vi "Insert Ramp Time Step Event.vi"(0 "VISA resource name":refnum<visa-resource-name>, 1 "Unit Address (1)":i16=1, 2 "Wait For Event (0: No)":u16(ring) items=["No", "Yes"], 5 "Current Step Number (1)":i16=1, 7 "Wait For Analog Inputs (0; 0; 0)":u16[](array[ring])=[0, 0, 0] items=["Don't Wait", "Wait For Analog Input"], 9 "Analog Input Values (32.0; 32.0; 32.0)":dbl[](array[numeric])=[32.0, 32.0, 32.0] format="%.2f", 11 "error in (no error)":errorcluster {"code" format="%.0x"}, 12 "Event Outputs (0; 0; 0; 0; 0; 0; 0; 0)":u16[](array[ring])=[0, 0, 0, 0, 0, 0, 0, 0] items=["Off", "On"], 13 "Wait For Event Inputs (0; 0; 0; 0)":u16[](array[ring])=[0, 0, 0, 0] items=["Don't Wait", "Wait For Off", "Wait For On"]) -> (4 "VISA resource name out":refnum<visa-resource-name>, 15 "error out":errorcluster {"code" format="%.0x"})   [LabVIEW 2010]
doc: "This is first part of two VIs, that inserts Ramp Time Step. This VI sets event inputs and outputs.\n\nNote: For correct function VIs MUST be activated in this sequence:\n1. WLF4 Insert Ramp Time Step Event.vi\n2. WLF4 Insert Ramp Time Step.vi"
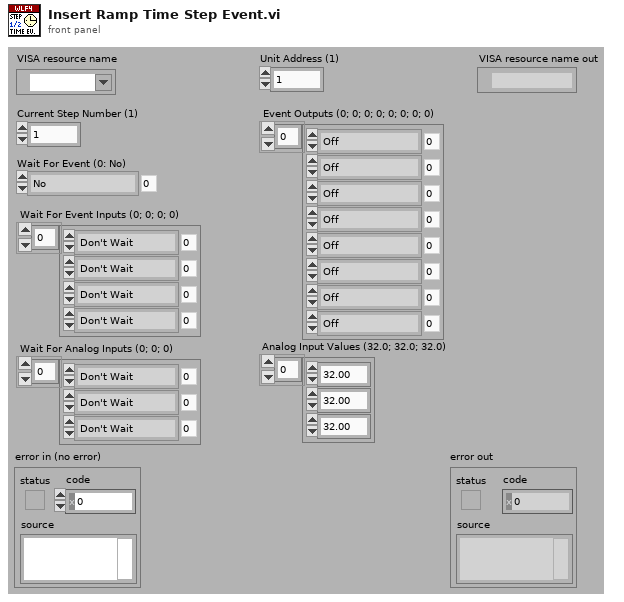
[diagram p1: front panel]
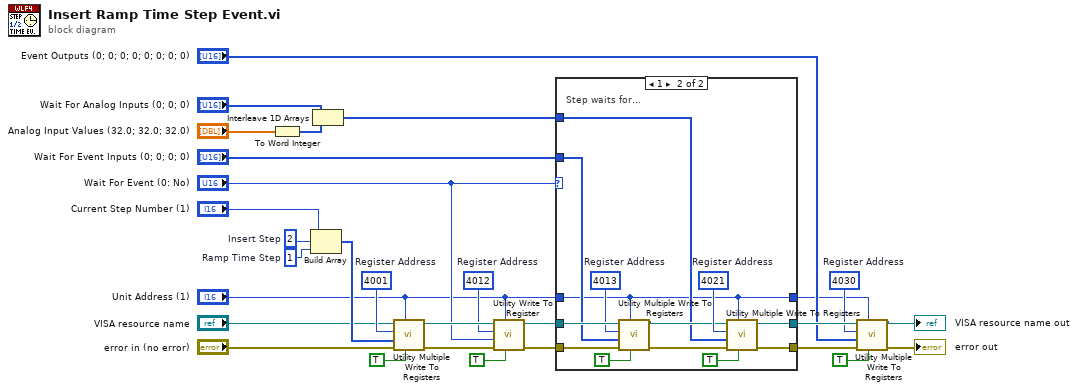
[diagram p0: block diagram]
diagram:
  w7 = 1  # Ramp Time Step
  w9 = u16 4030  # Register Address
  w21 = u16 4012  # Register Address
  w27 = u16 2  # Insert Step
  w29 = u16 4001  # Register Address
  n1 = To Word Integer(number="Analog Input Values (32.0; 32.0; 32.0)") -> (16bit integer=w14:i16[])
  n2 = Build Array("Current Step Number (1)", w27, w7) -> (w28:i32[])
  n3 = Interleave 1D Arrays("Wait For Analog Inputs (0; 0; 0)", w14) -> (w12:u16[])
  n4 = call "Utility Multiple Write To Registers.vi"("Direct Action?"=TRUE, "Unit Address (1)"="Unit Address (1)", "error in (no error)"="error in (no error)", "Array Of Data"=w28, "Register Address (0)"=w29, "VISA resource name"="VISA resource name") -> ("error out"=w23:errorcluster, "VISA resource name out"=w22:refnum<visa-resource-name>)  [unwired: 4 in]
  n5 = call "Utility Write To Register.vi"("Direct Action?"=TRUE, "Unit Address (1)"="Unit Address (1)", "error in (no error)"=w23, "Data (0)"="Wait For Event (0: No)", "Register Address (0)"=w21, "VISA resource name"=w22) -> ("error out"=w19:errorcluster, "VISA resource name out"=w20:refnum<visa-resource-name>)  [unwired: 4 in]
  n6 = case shown="1" "Wait For Event (0: No)" {
    tunnel: w20 -> [w32 w44]
    tunnel: w19 -> [w31 w45]
    tunnel: [w31 w37] -> w11
    tunnel: [w32 w36] -> w10
    tunnel: "Unit Address (1)" -> [w30 w35]
    tunnel: [w30 w35] -> w6
    tunnel: "Wait For Event Inputs (0; 0; 0; 0)" -> [_ w42]
    tunnel: w12 -> [_ w38]
    frame 0, Default {
      # "Step does not wait"
    }
    frame 1 {
      w41 = u16 4021  # Register Address
      w43 = u16 4013  # Register Address
      # "Step waits for..."
      n7 = call "Utility Multiple Write To Registers.vi"("Direct Action?"=TRUE, "Unit Address (1)"=w35, "error in (no error)"=w45, "Array Of Data"=w42, "Register Address (0)"=w43, "VISA resource name"=w44) -> ("error out"=w40:errorcluster, "VISA resource name out"=w39:refnum<visa-resource-name>)  [unwired: 4 in]
      n8 = call "Utility Multiple Write To Registers.vi"("Direct Action?"=TRUE, "Unit Address (1)"=w35, "error in (no error)"=w40, "Array Of Data"=w38, "Register Address (0)"=w41, "VISA resource name"=w39) -> ("error out"=w37:errorcluster, "VISA resource name out"=w36:refnum<visa-resource-name>)  [unwired: 4 in]
    }
  }
  n9 = call "Utility Multiple Write To Registers.vi"("Direct Action?"=TRUE, "Unit Address (1)"=w6, "error in (no error)"=w11, "Array Of Data"="Event Outputs (0; 0; 0; 0; 0; 0; 0; 0)", "Register Address (0)"=w9, "VISA resource name"=w10) -> ("error out"=→"error out":errorcluster, "VISA resource name out"=→"VISA resource name out":refnum<visa-resource-name>)  [unwired: 4 in]
